vi "Set Index.vi"(8 "error in (no error)":errorcluster, 10 "Index":u16, 11 "ODentry in":refnum<class "ODentry.lvclass">) -> (0 "error out":errorcluster, 3 "ODentry out":refnum<class "ODentry.lvclass">)   [LabVIEW 2024, in "EDS.lvlib" / "ODentry.lvclass"]
uses:
  ODentry.lvclass
  ODentry.lvclass/ODentry.ctl
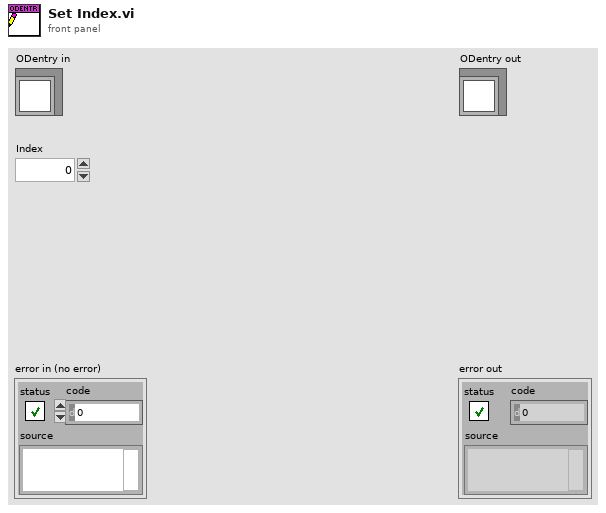
[diagram p1: front panel]
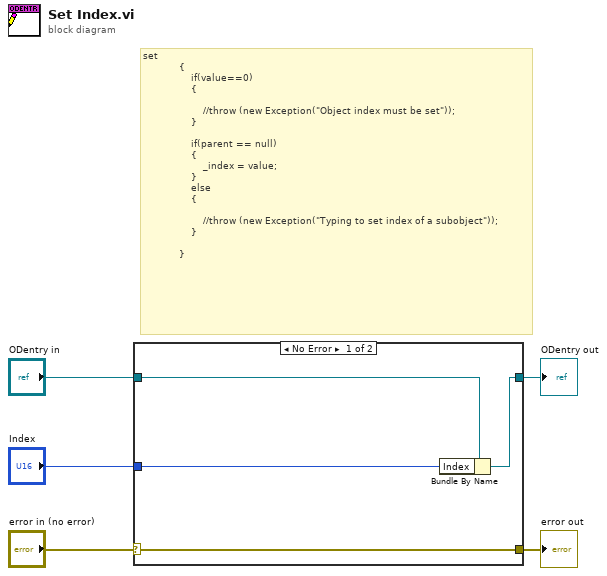
[diagram p0: block diagram]
diagram:
  # "set\n            {\n                if(value==0)\n                {\n\n                    //throw (new Exception(\"Object index must be set\"));\n                }\n\n                if(parent == null)\n                {\n                    _index = value;\n                }\n                else\n                {\n\n                    //throw (new Exception(\"Typing to set index of a subobject\"));\n                }\n               \n            }"
  n1 = case shown="No Error" "error in (no error)" {
    selector: "error in (no error)" -> [w9 w10]
    tunnel: [w9 w10] -> w4
    tunnel: [w7 w11] -> w2
    tunnel: "ODentry in" -> [w8 w11]
    tunnel: "Index" -> [w6 _]
    frame No Error {
      n2 = Bundle By Name(cluster=w8, "Index"=w6) -> (w7:refnum<class "ODentry.lvclass">)
    }
    frame Error {
    }
  }
  "error out" <- w4
  "ODentry out" <- w2
